vi "simulate_temperature.vi"(7 "Rauschfaktor":dbl, 9 "Schwankungen":dbl, 11 "Basiswert":dbl) -> (10 "Temperaturwert (°C)":dbl)   [LabVIEW 2025]
panel:
  in  "time":dbl
  out "Waveform Chart":dbl(graph)
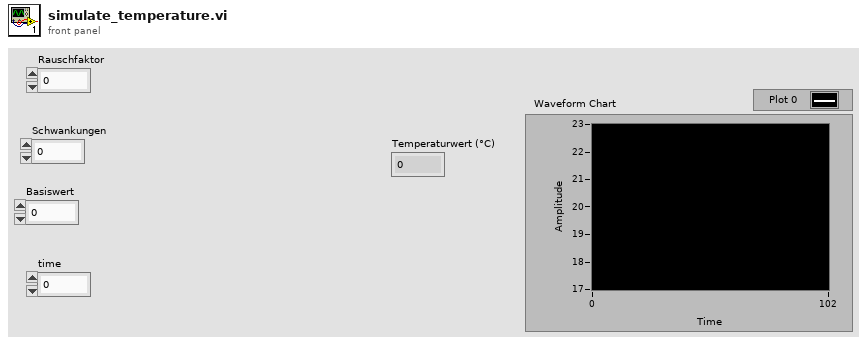
[diagram p1: front panel]
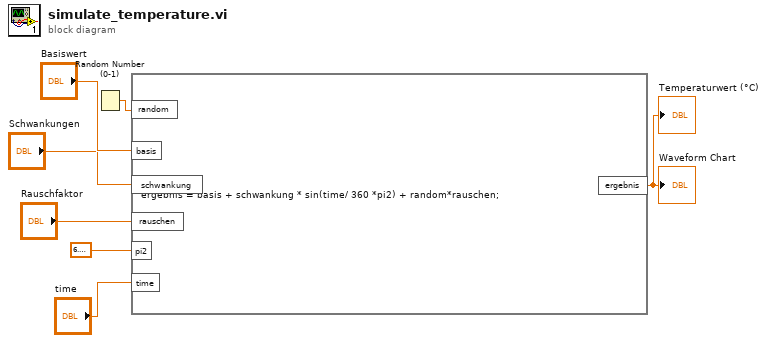
[diagram p0: block diagram]
diagram:
  n1 = Random Number (0-1)() -> (number: 0 to 1=w6:dbl)
  n2 = formula code="ergebnis = basis + schwankung * sin(time/ 360 *pi2) + random*rauschen;"("schwankung"="Schwankungen", "basis"="Basiswert", "rauschen"="Rauschfaktor", "pi2"=6.283185307179586, "random"=w6, "time"="time") -> ("ergebnis"=→"Temperaturwert (°C)" →"Waveform Chart":dbl)
